vi "generator-Lin-step.vi"(1 "step":i32, 2 "end":dbl, 3 "start":dbl) -> (0 "Array":dbl[](array[numeric]))   [LabVIEW 2021]
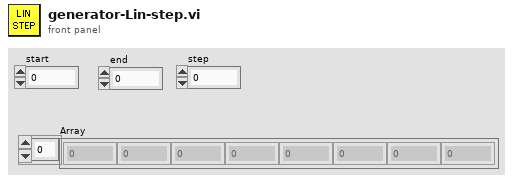
[diagram p1: front panel]
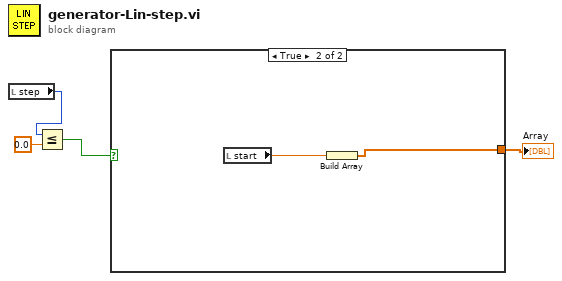
[diagram p0: block diagram]
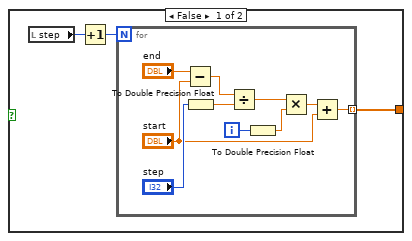
[diagram p2: hidden frame]
diagram:
  n1 = local read "step"() -> (w2:i32)
  n2 = Less Or Equal?(x=w2, y=0.0) -> (x <= y?=w1:bool)
  n3 = case shown="True" w1 {
    tunnel: [w5 w18] -> w4
    frame False {
      n4 = local read "step"() -> (w6:i32)
      n5 = Increment(x=w6) -> (x+1=w7:i32)
      n6 = for {
        N: w7 -> [_]
        tunnel: [w9] -> w5 mode=indexing
        i -> [w16]
        n7 = Subtract(x="end", y="start") -> (x-y=w17:dbl)
        n8 = To Double Precision Float(number="step") -> (double precision float=w15:dbl)
        n9 = Divide(x=w17, y=w15) -> (x/y=w13:dbl)
        n10 = To Double Precision Float(number=w16) -> (double precision float=w12:dbl)
        n11 = Multiply(x=w13, y=w12) -> (x*y=w11:dbl)
        n12 = Add(x=w11, y="start") -> (x+y=w9:dbl)
      }
    }
    frame True {
      n13 = local read "start"() -> (w19:dbl)
      n14 = Build Array(w19) -> (w18:dbl[])
    }
  }
  "Array" <- w4
